vi "Error Code HandlerSD.vi"(3 "DLL error code":u32) -> (0 "error out":errorcluster, 1 "dup DLL error code":u32)   [LabVIEW 2015]
doc: "Checks the return value received from an SDK DLL function call, here referred to as the <B>DLL error code</B>, and produces a standard LabVIEW error cluster that represents that error (or non-error).\n\nThe DLL error code DRV_SUCCESS is considered a non-error. All other DLL error codes are considered errors.\n\n<B>error out</B>'s integer member <B>code</B> is offset from the original DLL error code according to the Error Code Offset (or ECO) values stored in the <B>Error Code Offset global.vi</B> global variable.\n\n<B>error out</B>'s string member <B>source</B> contains the joined call chain string described in detail in <B>Get Error Source.vi</B>."
uses:
  Error Code Enum typedef.ctl
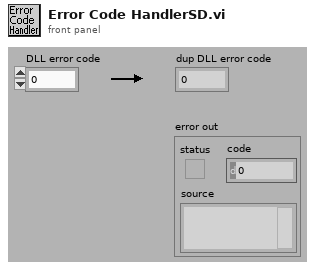
[diagram p1: front panel]
types:
  T1 = typedef "Error Code Enum typedef.ctl" = enum32{"N/A (0)", "DRV_ERROR_CODES", "DRV_SUCCESS", "DRV_VXDNOTINSTALLED", "DRV_ERROR_SCAN", "DRV_ERROR_CHECK_SUM", "DRV_ERROR_FILELOAD", "DRV_UNKNOWN_FUNC", "DRV_ERROR_VXD_INIT", "DRV_ERROR_ADDRESS", "DRV_ERROR_PAGELOCK", "DRV_ERROR_PAGEUNLOCK", "DRV_ERROR_BOARDTEST", "DRV_ERROR_ACK", "DRV_ERROR_UP_FIFO", "DRV_ERROR_PATTERN", "N/A (16)", "DRV_ACQUISITION_ERRORS", "DRV_ACQ_BUFFER", "DRV_ACQ_DOWNFIFO_FULL", "DRV_PROC_UNKONWN_INSTRUCTION", "DRV_ILLEGAL_OP_CODE", "DRV_KINETIC_TIME_NOT_MET", "DRV_ACCUM_TIME_NOT_MET", "DRV_NO_NEW_DATA", "N/A (25)", "DRV_SPOOLERROR", "N/A (27)", "N/A (28)", "N/A (29)", "N/A (30)", "N/A (31)", "N/A (32)", "DRV_TEMPERATURE_CODES", "DRV_TEMPERATURE_OFF", "DRV_TEMPERATURE_NOT_STABILIZED", "DRV_TEMPERATURE_STABILIZED", "DRV_TEMPERATURE_NOT_REACHED", "DRV_TEMPERATURE_OUT_RANGE", "DRV_TEMPERATURE_NOT_SUPPORTED", "DRV_TEMPERATURE_DRIFT", "N/A (41)", "N/A (42)", "N/A (43)", "N/A (44)", "N/A (45)", "N/A (46)", "N/A (47)", "N/A (48)", "DRV_GENERAL_ERRORS", "DRV_INVALID_AUX", "DRV_COF_NOTLOADED", "DRV_FPGAPROG", "DRV_FLEXERROR", "DRV_GPIBERROR", "N/A (55)", "N/A (56)", "N/A (57)", "N/A (58)", "N/A (59)", "N/A (60)", "N/A (61)", "N/A (62)", "N/A (63)", "DRV_DATATYPE", "DRV_DRIVER_ERRORS", "DRV_P1INVALID", "DRV_P2INVALID", "DRV_P3INVALID", "DRV_P4INVALID", "DRV_INIERROR", "DRV_COFERROR", "DRV_ACQUIRING", "DRV_IDLE", "DRV_TEMPCYCLE", "DRV_NOT_INITIALIZED", "DRV_P5INVALID", "DRV_P6INVALID", "DRV_INVALID_MODE", "DRV_INVALID_FILTER", "DRV_I2CERRORS", "DRV_I2CDEVNOTFOUND", "DRV_I2CTIMEOUT", "DRV_P7INVALID", "N/A (84)", "N/A (85)", "N/A (86)", "N/A (87)", "N/A (88)", "N/A (89)", "DRV_IOCERROR", "DRV_VRMVERSIONERROR"}
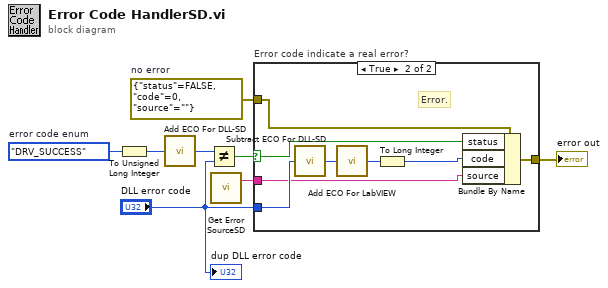
[diagram p0: block diagram]
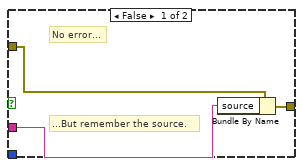
[diagram p2: hidden frame]
diagram:
  w2 = Error_Code_Enum_typedef."DRV_SUCCESS"  # error code enum
  w6 = errorcluster {"status"=FALSE, "code"=0, "source"=""}  # no error
  n1 = To Unsigned Long Integer(number=w2) -> (unsigned 32bit integer=w3:u32)
  n2 = call "Add ECO For DLL-SD.vi"("x"=w3) -> ("x + ECO4DLL"=w4:u32)
  n3 = Not Equal?(x=w4, y="DLL error code") -> (x != y?=w8:bool)
  n4 = call "Get Error SourceSD.vi"() -> ("error source"=w1:string)  [unwired: 2 in, 1 out]
  n5 = case "Error code indicate a real error?" shown="True" w8 {
    selector: w8 -> [_ w17]
    tunnel: [w11 w19] -> w7
    tunnel: w6 -> [w10 w18]
    tunnel: "DLL error code" -> [_ w15]
    tunnel: w1 -> [w9 w12]
    frame False {
      # "...But remember the source."
      # "No error..."
      n6 = Bundle By Name(cluster=w10, "source"=w9) -> (w11:errorcluster)
    }
    frame True {
      # "Error."
      n7 = call "Subtract ECO For DLL-SD.vi"("x"=w15) -> ("x - ECO4DLL"=w14:u32)
      n8 = call "Add ECO For LabVIEW.vi"("x"=w14) -> ("x + ECO4LabVIEW"=w16:u32)
      n9 = To Long Integer(number=w16) -> (32bit integer=w13:i32)
      n10 = Bundle By Name(cluster=w18, "status"=w17, "code"=w13, "source"=w12) -> (w19:errorcluster)
    }
  }
  "error out" <- w7
  "dup DLL error code" <- "DLL error code"
